vi "Get Buffer.vi"(11 "AI Voltage DAQmx Cont CFG in":refnum<class "AI Voltage DAQmx Cont CFG.lvclass">) -> (2 "Buffer Lossless DBL":refnum<class "Buffer Lossless DBL.lvclass">, 3 "AI Voltage DAQmx Cont CFG out":refnum<class "AI Voltage DAQmx Cont CFG.lvclass">)   [LabVIEW 2024, in "AI Voltage DAQmx Cont CFG.lvclass"]
uses:
  AI Voltage DAQmx Cont CFG.lvclass
  AI Voltage DAQmx Cont CFG.lvclass/AI Voltage DAQmx Cont CFG.ctl
  Buffers/Buffer Lossless DBL/Buffer Lossless DBL.lvclass
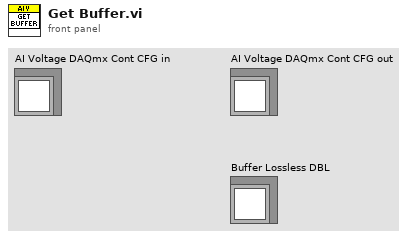
[diagram p1: front panel]
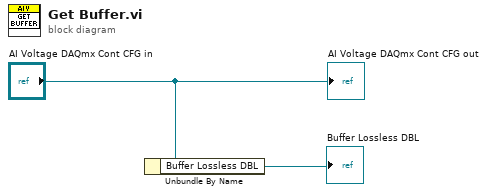
[diagram p0: block diagram]
diagram:
  n1 = Unbundle By Name("AI Voltage DAQmx Cont CFG in") -> ("Buffer Lossless DBL"=→"Buffer Lossless DBL":refnum<class "Buffer Lossless DBL.lvclass">)
  "AI Voltage DAQmx Cont CFG out" <- "AI Voltage DAQmx Cont CFG in"
